vi "receive message.vi"(8 "error in (no error)":errorcluster, 11 "Server in":refnum<class "Server.lvclass">) -> (0 "error out":errorcluster, 3 "Server out":refnum<class "Server.lvclass">)   [LabVIEW 2018, in "Server.lvclass"]
uses:
  Server.lvclass
  Server.lvclass/Server.ctl
  RxTx/CCS_RxTx.lvclass
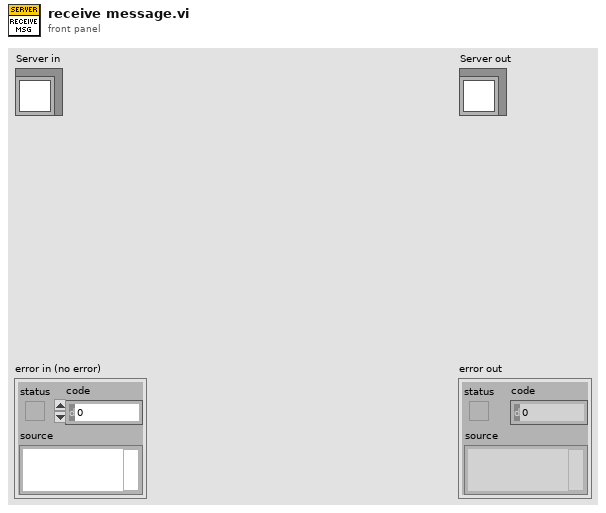
[diagram p1: front panel]
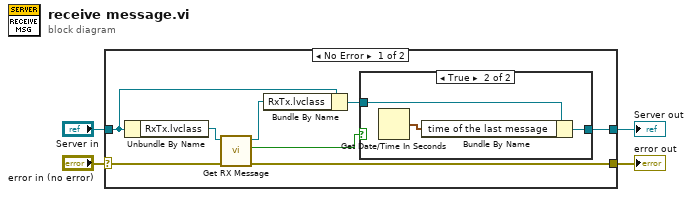
[diagram p0: block diagram]
diagram:
  n1 = case shown="No Error" "error in (no error)" {
    selector: "error in (no error)" -> [w11 w18]
    tunnel: [w9 w18] -> w3
    tunnel: [w10 w17] -> w1
    tunnel: "Server in" -> [w8 w17]
    frame No Error {
      n2 = Unbundle By Name(w8) -> ("RxTx.lvclass"=w12:refnum<class "CCS_RxTx.lvclass">)
      n3 = call "Get RX Message.vi"("error in (no error)"=w11, "RxTx in"=w12) -> ("error out"=w9:errorcluster, "new msg"=w5:bool, "RxTx out"=w6:refnum<class "CCS_RxTx.lvclass">)  [unwired: 7 in]
      n4 = Bundle By Name(cluster=w8, "RxTx.lvclass"=w6) -> (w7:refnum<class "Server.lvclass">)
      n5 = case shown="True" w5 {
        tunnel: w7 -> [w13 w16]
        tunnel: [w13 w15] -> w10
        frame False {
        }
        frame True {
          n6 = Get Date/Time In Seconds() -> (seconds since 1Jan1904=w14:timestamp)
          n7 = Bundle By Name(cluster=w16, "time of the last message"=w14) -> (w15:refnum<class "Server.lvclass">)
        }
      }
    }
    frame Error {
    }
  }
  "error out" <- w3
  "Server out" <- w1
